vi "WaitSingle.vi"(7 "wait option? (MoveDone)":i32(ring)=1 items=["InPosition", "MoveDone"], 8 "error in (no error)":errorcluster, 9 "timeout? (-1)":i32=-1, 10 "axis name":string, 11 "controller in":refnum<k24>) -> (0 "error out":errorcluster, 2 "completed":bool, 3 "controller out":refnum<k24>)   [LabVIEW 2013]
uses:
  C:/GEECS/Developers Version/source/Device Driver/AerotechStage/Sample Vis/Bin/Aerotech.Ensemble.dll
  Bin/Aerotech.Ensemble.dll
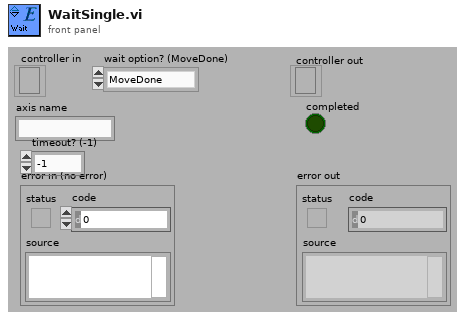
[diagram p1: front panel]
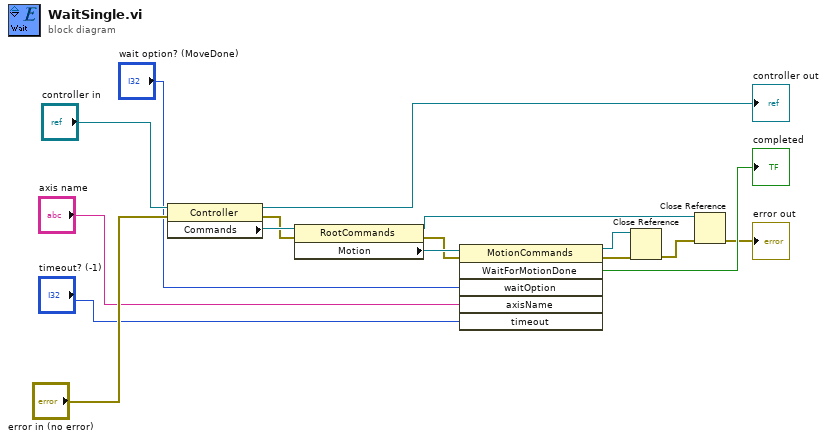
[diagram p0: block diagram]
diagram:
  n1 = property class="Controller"(reference="controller in", error in="error in (no error)") -> (reference out=→"controller out":refnum<k24>, error out=w11:errorcluster, "Commands"=w13:refnum<k24>)
  n2 = property class="RootCommands"(reference=w13, error in=w11) -> (reference out=w1:refnum<k24>, error out=w10:errorcluster, "Motion"=w12:refnum<k24>)
  n3 = invoke class="MotionCommands" method="WaitForMotionDone"(reference=w12, error in=w10, "waitOption"="wait option? (MoveDone)", "axisName"="axis name", "timeout"="timeout? (-1)") -> (reference out=w2:refnum<k24>, error out=w5:errorcluster, "WaitForMotionDone"=→"completed":bool)  [unwired: 1 in, 3 out]
  n4 = Close Reference(reference=w2, error in (no error)=w5) -> (error out=w3:errorcluster)
  n5 = Close Reference(reference=w1, error in (no error)=w3) -> (error out=→"error out":errorcluster)
